vi "Dashboard Main.vi"() -> ()   [LabVIEW 2011]
uses:
  <vilib>/Rock Robotics/WPI/DriverStation/WPI_DriverStationDigitalData.ctl
  DStoPCPacketTypeDef.ctl
panel:
  out "8 -- Battery":sgl(graph)
  out "Analog Input":sgl[](array[slide]) scale=0.0..5.0
  in  "Viewer":enum32{"Camera Image", "Kinect Skeleton"}(tab)
  in  "Video Enable":bool=TRUE
  out "Camera Image":T1(plugin-control)
  out "Buttons 1":cluster{"1":bool, "2":bool, "3":bool}
  out "Kinect 1":cluster{"X":dbl, "Y":dbl, "Z":dbl} {"X" scale=1.0..-1.0; "Y" scale=1.0..-1.0; "Z" scale=1.0..-1.0}
  out "Buttons 2":cluster{"1":bool, "2":bool, "3":bool}
  out "Kinect 2":cluster{"X":dbl, "Y":dbl, "Z":dbl} {"X" scale=1.0..-1.0; "Y" scale=1.0..-1.0; "Z" scale=1.0..-1.0}
  out "Version":string
  out "Skeleton Picture":picture
  out "Players":i8
  out "Dashboard Datatype Warning":string="Warning: The Dashboard Datatype used by the robot project and this dashboard do not match.\nSee diagram for more details."
  out "Robot IP Address":string
  out "Image Error Message":string="Timeout in Camera Communications"
  out "Solenoid Output":bool[](array[boolean])
  out "PWM":cluster{u8, u8}[](array[slide])=[{0, 157}, {0, 157}, {0, 157}, {0, 157}, {0, 157}, {0, 157}, {0, 157}, {0, 157}, {0, 157}, {0, 169}] scale=1.0..255.0
  out "GPIO Output Enable":bool[](array[boolean])
  out "GPIO State":bool[](array[boolean])
  out "Relay":cluster{"Forward":bool[], "Reverse":bool[]}
  # "Direction"
  # "Analog #1"
  # "1"
  # "7"
  # "Communications"
  # "Solenoid #1"
  # "1"
  # "8"
  # "Digital #1"
  # "1"
  # "10"
  # "1"
  # "14"
  # "1"
  # "8"
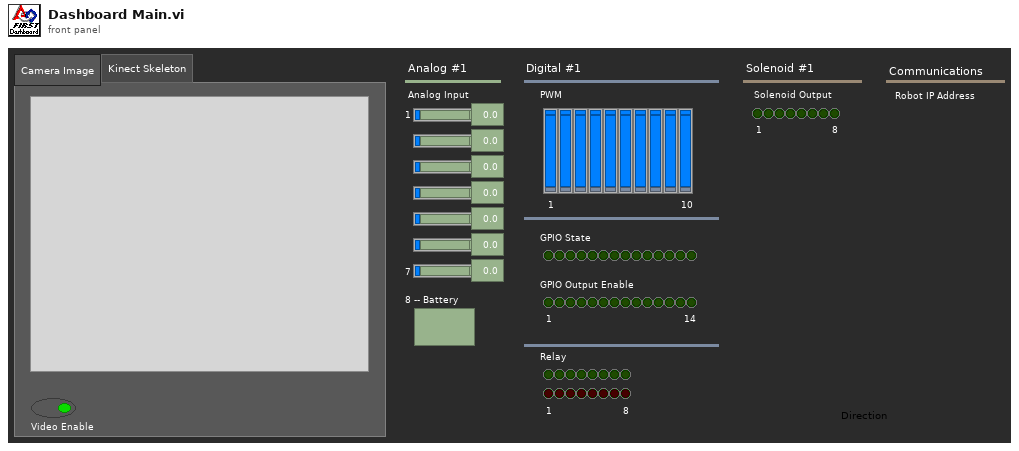
[diagram p1: front panel]
types:
  T1 = typedef "IMAQ Image.ctl" = refnum<image>
  T2 = typedef "WPI_DriverStationDigitalData.ctl" = cluster{"Relay Fwd":u8, "Relay Rev":u8, "GPIO":u16, "GPIO_OE":u16, "PWM":cluster{"PWM[0]":u8, "PWM[1]":u8, "PWM[2]":u8, "PWM[3]":u8, "PWM[4]":u8, "PWM[5]":u8, "PWM[6]":u8, "PWM[7]":u8, "PWM[8]":u8, "PWM[9]":u8}}
  T3 = typedef "DStoPCPacketTypeDef.ctl" = cluster{"Packet Index":u16, "Digital Inputs":u8, "Digital Out":u8, "Battery":u16, "Status":u8, "Error":u8, "Team ID":u16, "VersionMonth1":u8, "VersionMonth2":u8, "VersionDay1":u8, "VersionDay2":u8, "VersionYear1":u8, "VersionYear2":u8, "Revision1":u8, "Revision2":u8, "UnusedBuffer":u32, "UnusedBuffer 2":u16, "Reply Packet #":u16, "SPEED":dbl}
  T4 = cluster{cluster{"AnalogModule[0]":cluster{"Channel[0]":sgl, "Channel[1]":sgl, "Channel[2]":sgl, "Channel[3]":sgl, "Channel[4]":sgl, "Channel[5]":sgl, "Channel[6]":sgl, "Channel[7]":sgl}, "AnalogModule[1]":cluster{"Channel[0]":sgl, "Channel[1]":sgl, "Channel[2]":sgl, "Channel[3]":sgl, "Channel[4]":sgl, "Channel[5]":sgl, "Channel[6]":sgl, "Channel[7]":sgl}}, cluster{"DigitalModule[0]":T2}, "Solenoid":u8, "DigitalModule[1]":T2, cluster{"AnalogModule[0]":cluster{"Channel[3]":sgl}, "AnalogModule[1]":cluster{"Channel[1]":sgl}, "Cluster":T3}}
  T5 = typedef "Image Type" = u32
  T6 = typedef "LVBoundsTypeDef.ctl" = cluster{"Width":u32, "Height":u32}
  T7 = typedef "SkeletonTrackState.ctl" = enum32{"NotTracked", "PositionOnly", "Tracked"}
  T8 = cluster{"TrackingState":u8[], "Position":cluster{"x":sgl, "y":sgl, "z":sgl}, cluster{"x":sgl, "y":sgl, "z":sgl, sgl}[], "TrackState":T7}
  T9 = cluster{cluster{"ScaledToPercentRange":dbl, "ScaledToPercentRange":dbl, "ScaledToPercentRange":dbl}, cluster{bool, bool, bool}}[]
  T10 = cluster{cluster{"ScaledToPercentRange":dbl, "ScaledToPercentRange":dbl, "ScaledToPercentRange":dbl}, cluster{bool, bool, bool}}
  T11 = cluster{"ScaledToPercentRange":dbl, "ScaledToPercentRange":dbl, "ScaledToPercentRange":dbl}
  T12 = typedef "LVRectTypeDef.ctl" = cluster{"left":i16, "top":i16, "right":i16, "bottom":i16}
  T13 = cluster{"Competition mode":bool, "Robot Link":bool, "Autonomous":bool, "Enabled":bool, "E-Stop":bool}
  T14 = cluster{"AnalogModule[0]":cluster{"Channel[0]":sgl, "Channel[1]":sgl, "Channel[2]":sgl, "Channel[3]":sgl, "Channel[4]":sgl, "Channel[5]":sgl, "Channel[6]":sgl, "Channel[7]":sgl}, "AnalogModule[1]":cluster{"Channel[0]":sgl, "Channel[1]":sgl, "Channel[2]":sgl, "Channel[3]":sgl, "Channel[4]":sgl, "Channel[5]":sgl, "Channel[6]":sgl, "Channel[7]":sgl}}
  T15 = cluster{"Channel[0]":sgl, "Channel[1]":sgl, "Channel[2]":sgl, "Channel[3]":sgl, "Channel[4]":sgl, "Channel[5]":sgl, "Channel[6]":sgl, "Channel[7]":sgl}[]
  T16 = cluster{"Channel[0]":sgl, "Channel[1]":sgl, "Channel[2]":sgl, "Channel[3]":sgl, "Channel[4]":sgl, "Channel[5]":sgl, "Channel[6]":sgl, "Channel[7]":sgl}
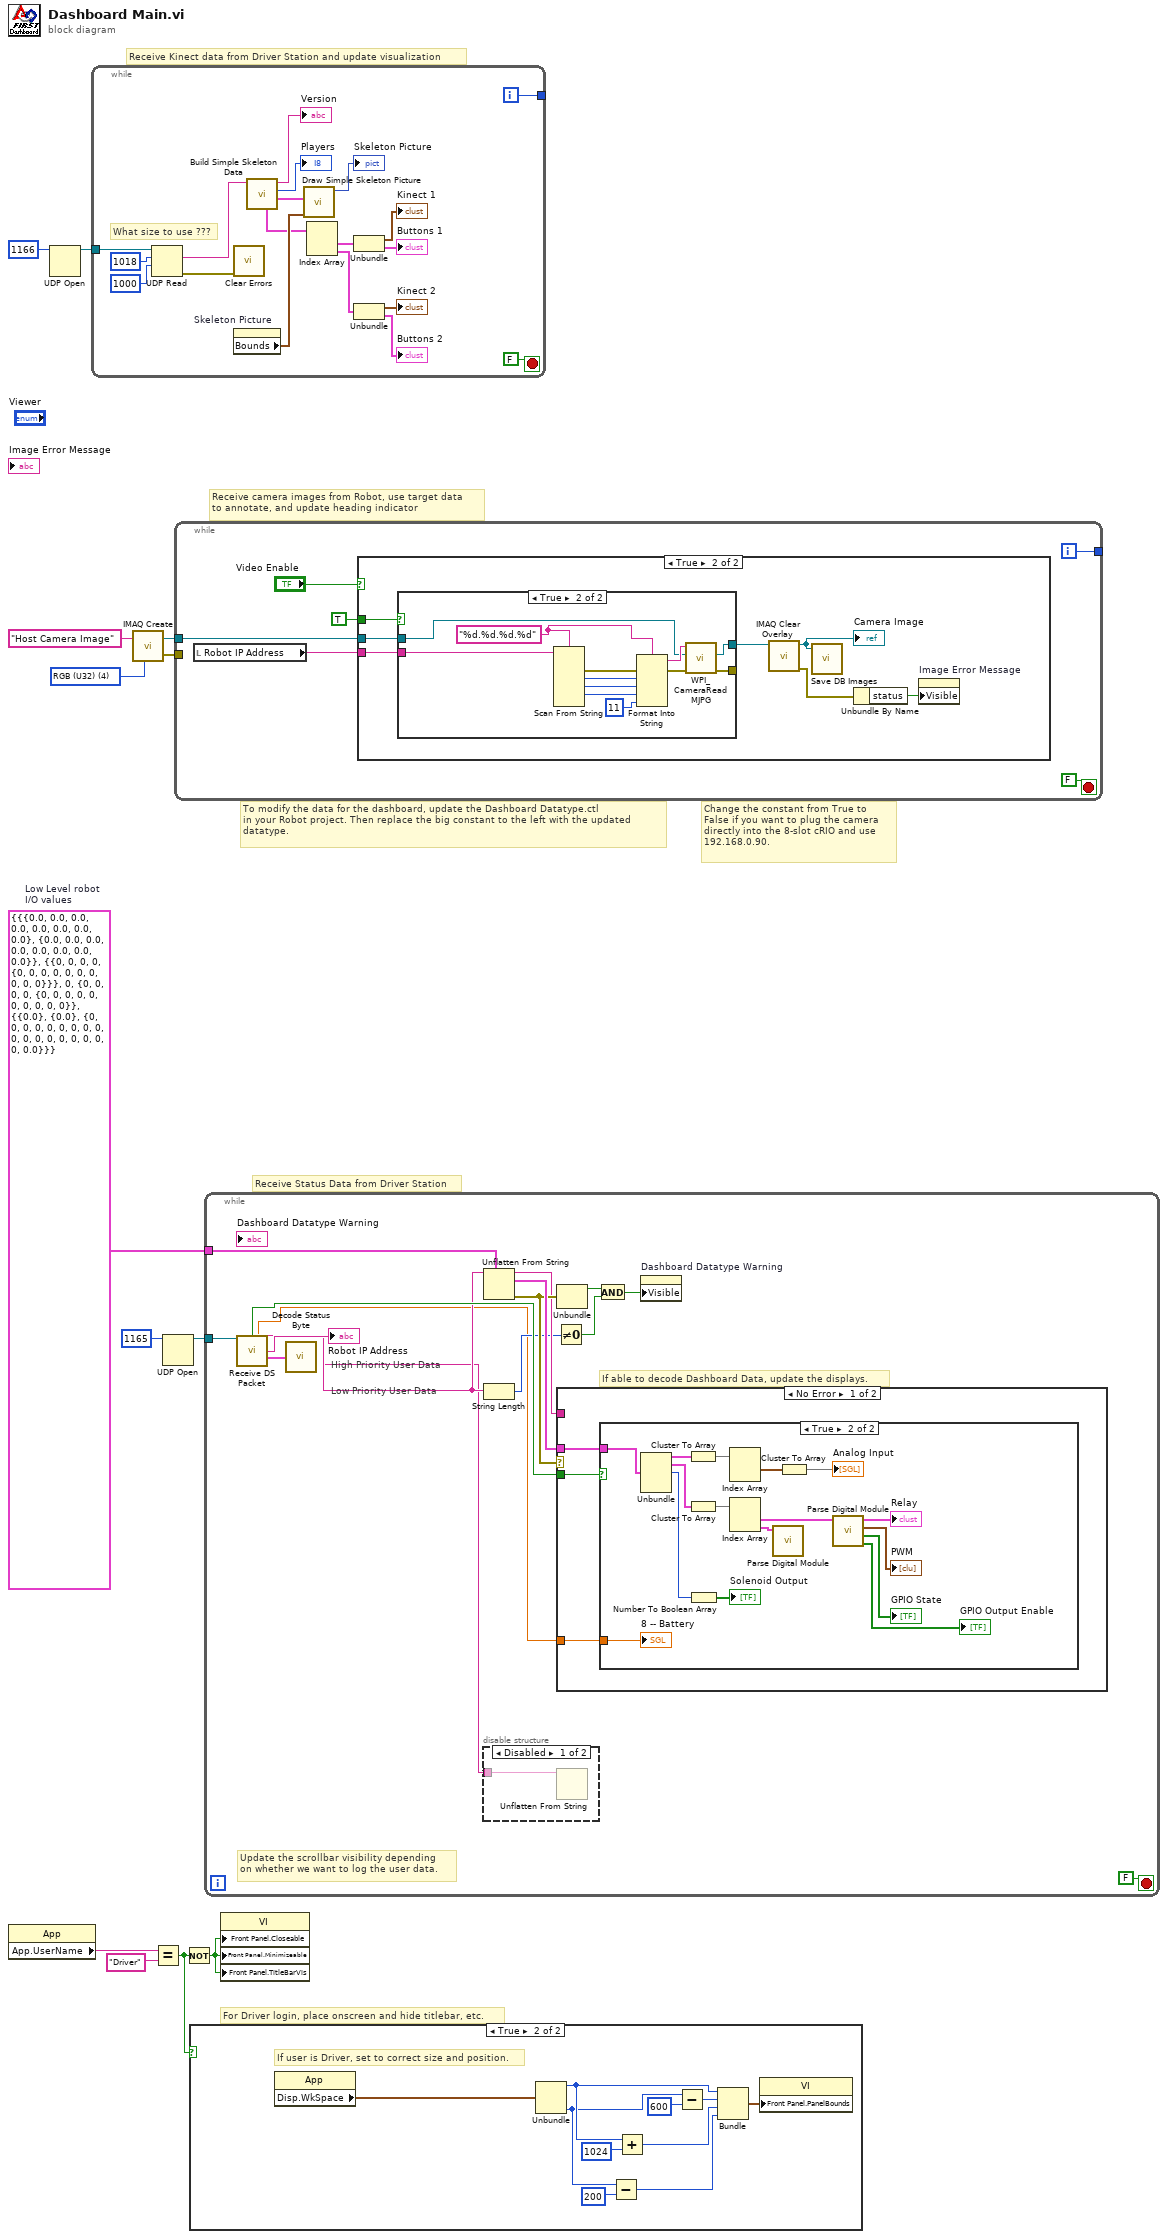
[diagram p0: block diagram]
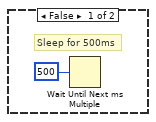
[diagram p6: hidden frame]
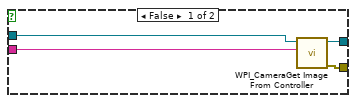
[diagram p7: hidden frame]
diagram:
  w3 = T4 {{"AnalogModule[0]"={"Channel[0]"=0.0, "Channel[1]"=0.0, "Channel[2]"=0.0, "Channel[3]"=0.0, "Channel[4]"=0.0, "Channel[5]"=0.0, "Channel[6]"=0.0, "Channel[7]"=0.0}, "AnalogModule[1]"={"Channel[0]"=0.0, "Channel[1]"=0.0, "Channel[2]"=0.0, "Channel[3]"=0.0, "Channel[4]"=0.0, "Channel[5]"=0.0, "Channel[6]"=0.0, "Channel[7]"=0.0}}, {"DigitalModule[0]"={"Relay Fwd"=0, "Relay Rev"=0, "GPIO"=0, "GPIO_OE"=0, "PWM"={"PWM[0]"=0, "PWM[1]"=0, "PWM[2]"=0, "PWM[3]"=0, "PWM[4]"=0, "PWM[5]"=0, "PWM[6]"=0, "PWM[7]"=0, "PWM[8]"=0, "PWM[9]"=0}}}, "Solenoid"=0, "DigitalModule[1]"={"Relay Fwd"=0, "Relay Rev"=0, "GPIO"=0, "GPIO_OE"=0, "PWM"={"PWM[0]"=0, "PWM[1]"=0, "PWM[2]"=0, "PWM[3]"=0, "PWM[4]"=0, "PWM[5]"=0, "PWM[6]"=0, "PWM[7]"=0, "PWM[8]"=0, "PWM[9]"=0}}, {"AnalogModule[0]"={"Channel[3]"=0.0}, "AnalogModule[1]"={"Channel[1]"=0.0}, "Cluster"={"Packet Index"=0, "Digital Inputs"=0, "Digital Out"=0, "Battery"=0, "Status"=0, "Error"=0, "Team ID"=0, "VersionMonth1"=0, "VersionMonth2"=0, "VersionDay1"=0, "VersionDay2"=0, "VersionYear1"=0, "VersionYear2"=0, "Revision1"=0, "Revision2"=0, "UnusedBuffer"=0, "UnusedBuffer 2"=0, "Reply Packet #"=0, "SPEED"=0.0}}}  # Low Level robot I/O values
  w11 = T5 4 items=["Grayscale (U8)", "Grayscale (I16)", "Grayscale (SGL)", "Complex (CSG)", "RGB (U32)", "HSL (U32)", "RGB (U64)"] ("Image Type")
  # "Change the constant from True to\nFalse if you want to plug the camera\ndirectly into the 8-slot cRIO and use\n192.168.0.90."
  # "Receive Kinect data from Driver Station and update visualization"
  # "For Driver login, place onscreen and hide titlebar, etc."
  # "To modify the data for the dashboard, update the Dashboard Datatype.ctl\nin your Robot project. Then replace the big constant to the left with the updated\ndatatype."
  # "Receive Status Data from Driver Station"
  # "Receive camera images from Robot, use target data\nto annotate, and update heading indicator"
  n1 = property class="App"() -> ("App.UserName"=w6:string)  [unwired: 2 in, 2 out]
  n2 = UDP Open(11:u16 1166 ("port")) -> (port=w1:refnum<k16>)  [unwired: 2 in, 4 out]
  n3 = while {
    tunnel: w1 -> [w30]
    tunnel: [w14] -> _
    i -> [w14]
    stop <- FALSE stop-if-true
    # "What size to use ???"
    n4 = UDP Read(connection ID=w30, max size (548)=1018 ("bytes to read"), timeout ms (25000)=1000) -> (data out=w24:string, error out=w22:errorcluster)  [unwired: 1 in, 3 out]
    n5 = call <vilib>:"Clear Errors.vi"("error in (no error)"=w22) -> ()  [unwired: 6 in, 1 out]
    n6 = property on="Skeleton Picture" class="Pict"() -> ("Bounds"=w26:T6)  [unwired: 2 in, 2 out]
    n7 = call "Build Simple Skeleton Data.vi"("data out"=w24) -> ("Skeleton Data"=w25:T8, "NumPlayers"=→"Players":i8, "Version String"=→"Version":string, "Simple Joystick Info"=w21:T9)  [unwired: 6 in, 1 out]
    n8 = call "Draw Simple Skeleton Picture.vi"("Bounds"=w26, "Simple Skeleton"=w25) -> ("new picture out"=→"Skeleton Picture":picture)  [unwired: 9 in]
    n9 = Index Array(array=w21) -> (element #1=w20:T10, element #2=w19:T10)  [unwired: 2 in]
    n10 = Unbundle(w20) -> (→"Kinect 1":T11, →"Buttons 1":cluster{bool, bool, bool})
    n11 = Unbundle(w19) -> (→"Kinect 2":T11, →"Buttons 2":cluster{bool, bool, bool})
  }
  n12 = call "IMAQ Create"("Image Name"="Host Camera Image", "Image Type"=w11) -> ("New Image"=w9:T1, "error out"=w8:errorcluster)  [unwired: 2 in, 1 out]
  n13 = Equal?(x=w6, y="Driver") -> (x = y?=w5:bool)
  n14 = UDP Open(11:u16 1165 ("port")) -> (port=w12:refnum<k16>)  [unwired: 2 in, 4 out]
  n15 = while {
    tunnel: w9 -> [w36]
    tunnel: w8 -> [_]
    tunnel: [w33] -> _
    i -> [w33]
    stop <- FALSE stop-if-true
    n16 = local read "Robot IP Address"() -> (w37:string)
    n17 = case shown="True" "Video Enable" {
      tunnel: w37 -> [_ w46]
      tunnel: w36 -> [_ w45]
      tunnel: TRUE -> [_ w40]
      frame False {
        # "Sleep for 500ms"
        n18 = Wait Until Next ms Multiple(millisecond multiple=u32 500) -> ()  [unwired: 1 out]
      }
      frame True {
        n19 = case shown="True" w40 {
          tunnel: w45 -> [w49 w56]
          tunnel: [w47 w54] -> _
          tunnel: [w48 w55] -> w42
          tunnel: w46 -> [w50 w59]
          frame False {
            n20 = call <vilib>:"WPI_CameraGet Image From Controller.vi"("Controller Address"=w50, "Image"=w49) -> ("error out"=w47:errorcluster, "Image Out"=w48:T1)  [unwired: 2 in, 6 out]
          }
          frame True {
            w51 = "%d.%d.%d.%d" ("format string")
            n21 = Scan From String(format string=w51, input string=w59) -> (error out=w58:errorcluster, output 1=w60:i32, output 2=w61:i32, output 3=w62:i32)  [unwired: 2 in, 7 out]
            n22 = Format Into String(format string=w51, error in=w58, w60, w61, w62, 11 ("IP Suffix:")) -> (resulting string=w57:string, error out=w53:errorcluster)  [unwired: 1 in]
            n23 = call <vilib>:"WPI_CameraRead MJPG.vi"("error in"=w53, "Image"=w56, "address"=w57) -> ("error out"=w54:errorcluster, "Image Out"=w55:T1)  [unwired: 7 in]
          }
        }
        n24 = call "IMAQ Clear Overlay"("Image"=w42) -> ("error out"=w43:errorcluster, "Image Out"=w41:T1)  [unwired: 2 in, 7 out]
        "Camera Image" <- w41
        n25 = call "Save DB Images.vi"("Image"=w41) -> ()  [unwired: 2 in, 1 out]
        n26 = Unbundle By Name(w43) -> ("status"=w44:bool)
        n27 = property on="Image Error Message" class="Str"("Visible"=w44) -> ()  [unwired: 2 in, 2 out]
      }
    }
  }
  n28 = Not(x=w5) -> (.not. x?=w4:bool)
  n29 = case shown="True" w5 {
    frame False {
    }
    frame True {
      # "If user is Driver, set to correct size and position."
      n30 = property class="App"() -> ("Disp.WkSpace"=w72:T12)  [unwired: 2 in, 2 out]
      n31 = Unbundle(w72) -> ("left"=w67:i16, "bottom"=w63:i16)  [unwired: 2 out]
      n32 = Subtract(x=w63, y=200) -> (x-y=w64:i32)
      n33 = Add(x=w67, y=1024) -> (x+y=w68:i32)
      n34 = Subtract(x=w63, y=600) -> (x-y=w69:i32)
      n35 = Bundle("left"=w67, w69, w68, w64) -> (w71:cluster{"left":i16, i32, i32, i32})  [unwired: 1 out]
      n36 = property class="VI"("Front Panel.PanelBounds"=w71) -> ()  [unwired: 2 in, 2 out]
    }
  }
  n37 = while {
    tunnel: w12 -> [w86]
    tunnel: w3 -> [w85]
    stop <- FALSE stop-if-true
    # "High Priority User Data"
    # "Low Priority User Data"
    # "Update the scrollbar visibility depending\non whether we want to log the user data."
    # "If able to decode Dashboard Data, update the displays."
    n38 = call "Receive DS Packet.vi"("Recv Socket"=w86) -> ("New Dashboard Data"=w82:bool, "Battery"=w73:sgl, "Robot IP Address"=→"Robot IP Address":string, "Status"=w87:T13, "Low Priority User Data"=w75:string, "High Priority User Data"=w74:string)  [unwired: 1 in, 8 out]
    n39 = call "Decode Status Byte.vi"("Status Byte"=w87) -> ()  [unwired: 2 out]
    n40 = Unflatten From String(type=w85, binary string=w75) -> (rest of the binary string=w78:string, value=w84:T4, error out=w83:errorcluster)  [unwired: 1 in, 2 out]
    n41 = String Length(string=w75) -> (length=w77:i32)
    n42 = disable-structure shown="Disabled" {
      disable-tunnel: w74 -> [w89 _]
      frame Disabled {
        n43 = Unflatten From String(binary string=w89) -> ()  [unwired: 2 in, 5 out]
      }
      frame Enabled {
      }
    }
    n44 = Not Equal To 0?(x=w77) -> (x != 0?=w80:bool)
    n45 = Unbundle(w83) -> ("status"=w79:bool)  [unwired: 2 out]
    n46 = case shown="No Error" w83 {
      tunnel: w84 -> [w92 _]
      tunnel: w82 -> [w91 _]
      tunnel: w78 -> [_ _]
      tunnel: w73 -> [w90 _]
      frame No Error {
        n47 = case shown="True" w91 {
          tunnel: w92 -> [_ w99]
          tunnel: w90 -> [_ w93]
          frame False {
            # "Don't update if the robot hasn't sent new data"
          }
          frame True {
            n48 = Unbundle(w99) -> (w96:T14, w97:cluster{"DigitalModule[0]":T2}, "Solenoid"=w98:u8)  [unwired: 2 out]
            n49 = Cluster To Array(cluster=w96) -> (array=w107:T15)
            n50 = Cluster To Array(cluster=w97) -> (array=w106:T2[])
            n51 = Number To Boolean Array(number=w98) -> (Boolean array=→"Solenoid Output":bool[])
            n52 = Index Array(array=w107) -> (element #1=w94:T16)  [unwired: 2 in, 1 out]
            n53 = Index Array(array=w106) -> (element #1=w105:T2, element #2=w100:T2)  [unwired: 2 in]
            n54 = call "Parse Digital Module.vi"("DigitalModule"=w100) -> ()  [unwired: 11 out]
            n55 = Cluster To Array(cluster=w94) -> (array=→"Analog Input":sgl[])
            n56 = call "Parse Digital Module.vi"("DigitalModule"=w105) -> ("GPIO Output Enable"=→"GPIO Output Enable":bool[], "GPIO State"=→"GPIO State":bool[], "PWM"=→"PWM":cluster{u8, u8}[], "Relay"=→"Relay":cluster{"Forward":bool[], "Reverse":bool[]})  [unwired: 7 out]
            "8 -- Battery" <- w93
          }
        }
      }
      frame Error {
        # "Your datatypes don't match. The Dashboard Datatype.ctl in your Robot project\nand the big constant to the left of the loop need to match."
      }
    }
    n57 = And(x=w79, y=w80) -> (x .and. y?=w81:bool)
    n58 = property on="Dashboard Datatype Warning" class="Str"("Visible"=w81) -> ()  [unwired: 2 in, 2 out]
  }
  n59 = property class="VI"("Front Panel.Closeable"=w4, "Front Panel.Minimizeable"=w4, "Front Panel.TitleBarVis"=w4) -> ()  [unwired: 2 in, 2 out]
